vi "Error Query.vi"(8 "error in (no error)":errorcluster, 11 "VISA resource name":refnum<visa-resource-name>) -> (0 "error out":errorcluster, 1 "Error Message":string, 2 "Error Code":i32[](array[numeric]), 3 "VISA resource name out":refnum<visa-resource-name>)   [LabVIEW 2013, in "HadCon.lvlib"]
doc: "Queries the instrument for any errors in the instrument's error queue. It will continue to read errors until all errors have been read from the instrument. Any errors will be returned in the <B>error out</B> control.\n\n<B>Note:</B>\nThis VI is called automatically by most driver VIs so it is not usually necessary to call this in an application."
uses:
  <instrlib>/HadCon/HadCon.lvlib
panel:
  # "EDIT: Note: The Error Query VI is included as a subVI in all driver VIs except low-level API VIs. If the instrument does not support error query, then remove the VI and remove subVI calls in each instrument driver VI that calls it."
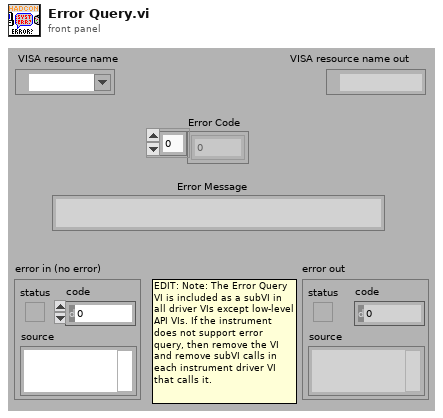
[diagram p1: front panel]
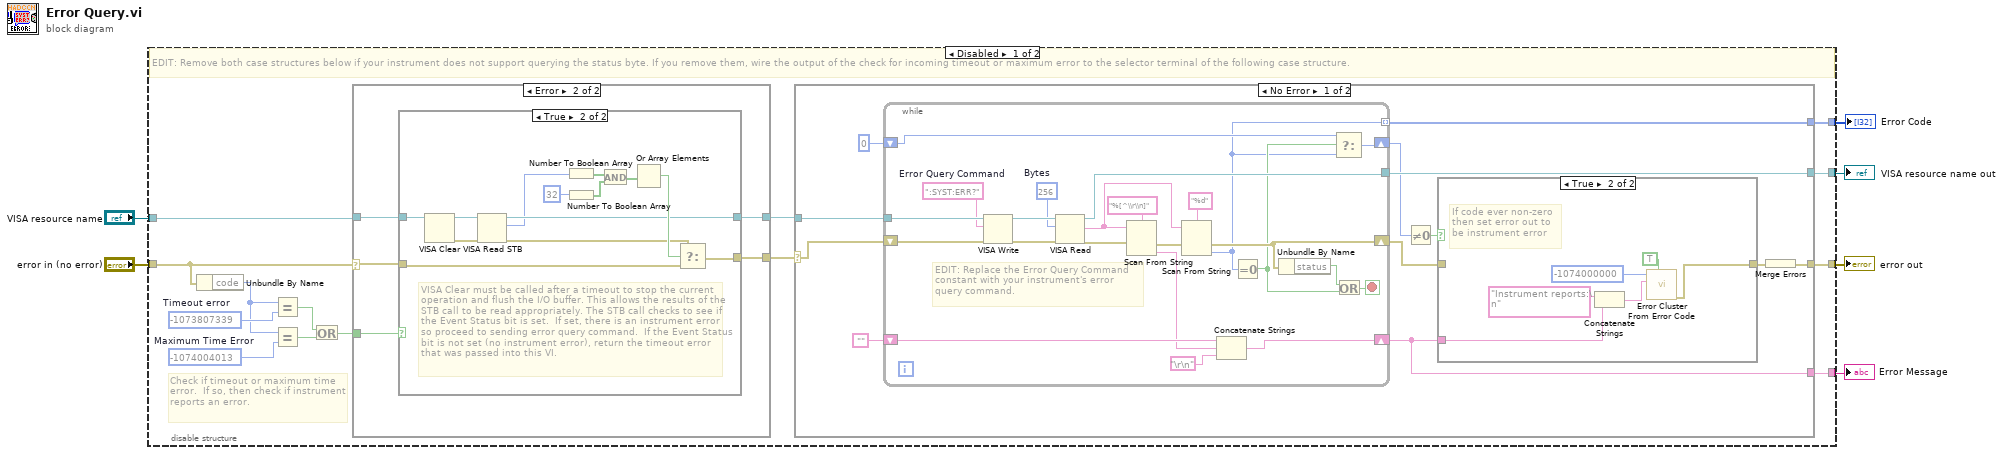
[diagram p0: block diagram]
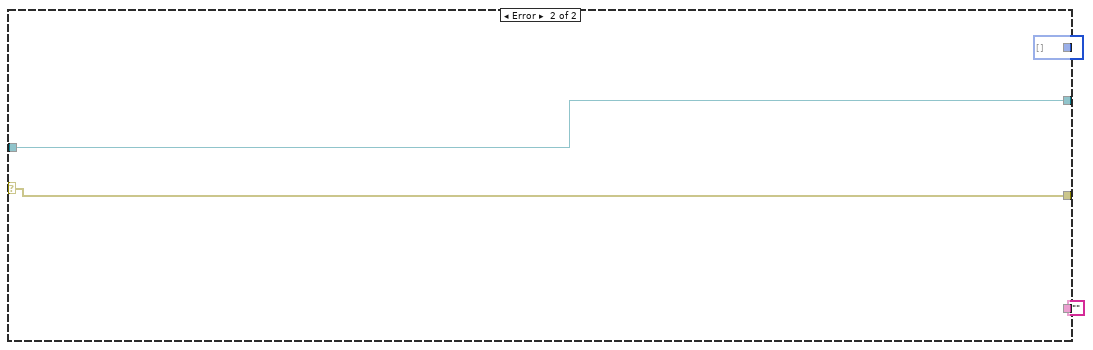
[diagram p5: hidden frame]
diagram:
  n1 = disable-structure shown="Disabled" {
    disable-tunnel: [w20 w89] -> w6
    disable-tunnel: [w19 w90] -> w5
    disable-tunnel: [w18 _] -> w4
    disable-tunnel: [w17 _] -> w3
    disable-tunnel: "VISA resource name" -> [w14 w89]
    disable-tunnel: "error in (no error)" -> [w7 w90]
    frame Disabled {
      w11 = -1074004013  # Maximum Time Error
      w13 = -1073807339  # Timeout error
      # "Check if timeout or maximum time error.  If so, then check if instrument reports an error."
      # "EDIT: Remove both case structures below if your instrument does not support querying the status byte. If you remove them, wire the output of the check for incoming timeout or maximum error to the selector terminal of the following case structure."
      n2 = Unbundle By Name(w7) -> ("code"=w12:i32)
      n3 = Equal?(x=w12, y=w13) -> (x = y?=w9:bool)
      n4 = Equal?(x=w12, y=w11) -> (x = y?=w10:bool)
      n5 = Or(x=w9, y=w10) -> (x .or. y?=w8:bool)
      n6 = case shown="Error" w7 {
        selector: w7 -> [w21 w25]
        tunnel: w14 -> [w22 w27]
        tunnel: [w22 w26] -> w15
        tunnel: [w21 w24] -> w16
        tunnel: w8 -> [_ w23]
        frame No Error {
        }
        frame Error {
          n7 = case shown="True" w23 {
            tunnel: w27 -> [w29 w35]
            tunnel: [w29 w32] -> w26
            tunnel: w25 -> [w28 w38]
            tunnel: [w28 w37] -> w24
            frame False {
              # "Error code not a timeout, so best to pass on to user."
            }
            frame True {
              # "VISA Clear must be called after a timeout to stop the current operation and flush the I/O buffer. This allows the results of the  STB call to be read appropriately. The STB call checks to see if the Event Status bit is set.  If set, there is an instrument error so proceed to sending error query command.  If the Event Status bit is not set (no instrument error), return the timeout error that was passed into this VI."
              n8 = VISA Clear(VISA resource name=w35) -> (VISA resource name out=w34:refnum<visa-resource-name>, error out=w33:errorcluster)  [unwired: 1 in]
              n9 = VISA Read STB(8:w33, 11:w34) -> (0:w31:errorcluster, 2:w30:u16, 3:w32:refnum<visa-resource-name>)
              n10 = Number To Boolean Array(number=w30) -> (Boolean array=w39:bool[])
              n11 = Number To Boolean Array(number=32) -> (Boolean array=w41:bool[])
              n12 = And(x=w39, y=w41) -> (x .and. y?=w40:bool[])
              n13 = Or Array Elements(Boolean array=w40) -> (logical OR=w36:bool)
              n14 = Select(t=w31, s=w36, f=w38) -> (s? t:f=w37:errorcluster)
            }
          }
        }
      }
      n15 = case shown="No Error" w16 {
        selector: w16 -> [w43 w85]
        tunnel: [w54 w88] -> w20
        tunnel: w15 -> [w53 w88]
        tunnel: [w51 w85] -> w19
        tunnel: [w46 ""] -> w18
        tunnel: [w45 i32[] []] -> w17
        frame No Error {
          n16 = while {
            tunnel: [w84] -> w54
            tunnel: w53 -> [w83]
            shift-right: [w71] -> w46
            shift-left: "" -> [w74]
            shift-right: [w69] -> w47
            shift-left: 0 -> [w70]
            shift-right: [w67] -> w44
            shift-left: w43 -> [w68]
            tunnel: [w62] -> w45 mode=indexing
            stop <- w77 stop-if-true
            w81 = u32 256  # Bytes
            w79 = ":SYST:ERR?"  # Error Query Command
            # "EDIT: Replace the Error Query Command\nconstant with your instrument's error\nquery command."
            n17 = VISA Write(VISA resource name=w83, write buffer=w79, error in (no error)=w68) -> (VISA resource name out=w82:refnum<visa-resource-name>, error out=w80:errorcluster)  [unwired: 1 out]
            n18 = VISA Read(VISA resource name=w82, byte count=w81, error in (no error)=w80) -> (VISA resource name out=w84:refnum<visa-resource-name>, read buffer=w75:string, error out=w66:errorcluster)  [unwired: 1 out]
            n19 = Scan From String(format string="%[^\\r\\n]", input string=w75, error in=w66) -> (error out=w65:errorcluster, output 1=w72:string)  [unwired: 2 in, 2 out]
            n20 = Scan From String(format string="%d", input string=w75, error in=w65) -> (error out=w67:errorcluster, output 1=w62:i32)  [unwired: 2 in, 2 out]
            n21 = Concatenate Strings(w74, w72, "\r\n") -> (w71:string)
            n22 = Equal To 0?(x=w62) -> (x = 0?=w63:bool)
            n23 = Unbundle By Name(w67) -> ("status"=w64:bool)
            n24 = Select(t=w70, s=w63, f=w62) -> (s? t:f=w69:i32)
            n25 = Or(x=w64, y=w63) -> (x .or. y?=w77:bool)
          }
          n26 = Not Equal To 0?(x=w47) -> (x != 0?=w49:bool)
          n27 = case shown="True" w49 {
            tunnel: w46 -> [_ w60]
            tunnel: [w55 w56] -> w48
            tunnel: w44 -> [w55 _]
            frame False {
            }
            frame True {
              # "If code ever non-zero\nthen set error out to\nbe instrument error"
              n28 = Concatenate Strings("Instrument reports:\n" ("Source"), w60) -> (w57:string)
              n29 = call <vilib>:"Error Cluster From Error Code.vi"("show call chain? (False)"=TRUE, "error message (\"\")"=w57, "error code (0)"=-1074000000 ("Code")) -> ("error out"=w56:errorcluster)  [unwired: 6 in]
            }
          }
          n30 = Merge Errors(w48) -> (w51:errorcluster)
        }
        frame Error {
        }
      }
    }
    frame Enabled {
    }
  }
  "VISA resource name out" <- w6
  "error out" <- w5
  "Error Message" <- w4
  "Error Code" <- w3
